vi "N-664 Test Panel.vi"() -> ()   [LabVIEW 2020]
uses:
  <vilib>/Instr/_visa.llb/VISA Configure Serial Port (Instr).vi
panel:
  out "Latest Error":errorcluster
  in  "COM Port":refnum<visa-resource-name>
  in  "Quit":bool
  out "Reply":string
  in  "Send Command":bool
  in  "Command":string
  # "*IDN? - Get device info"
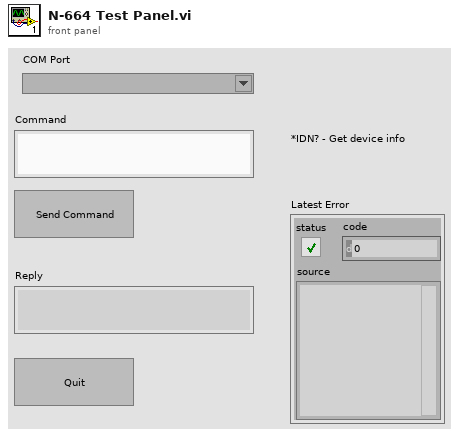
[diagram p1: front panel]
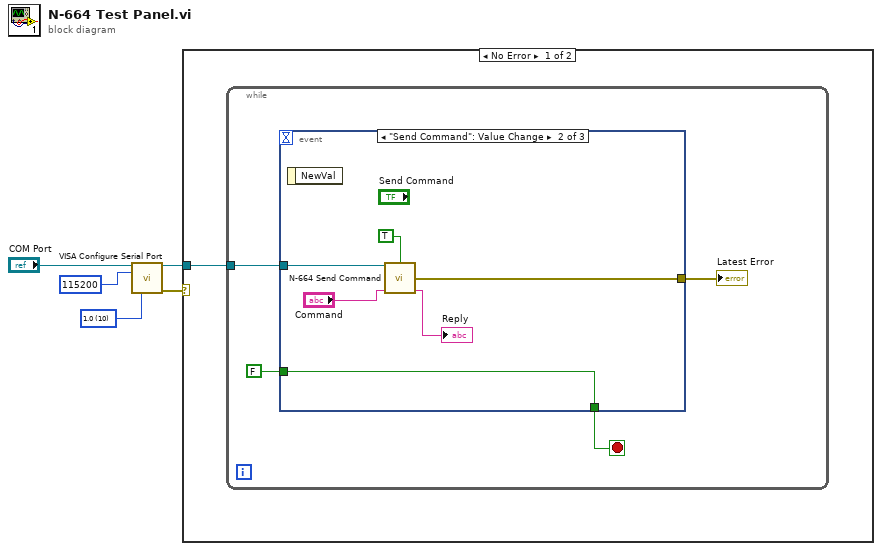
[diagram p0: block diagram]
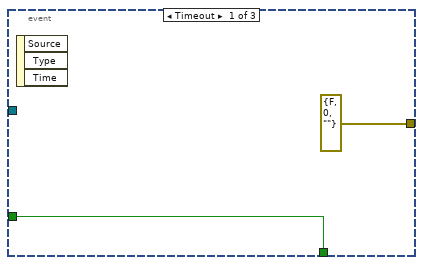
[diagram p2: hidden frame]
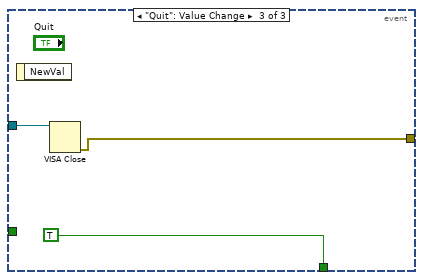
[diagram p3: hidden frame]
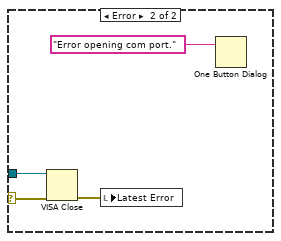
[diagram p4: hidden frame]
diagram:
  w5 = u16 10 items=["1.0"=10, "1.5"=15, "2.0"=20] ("stop bits (10: 1 bit)")
  n1 = call-poly "VISA Configure Serial Port"("VISA resource name"="COM Port", "baud rate (9600)"=u32 115200, "stop bits (10: 1 bit)"=w5) -> ("VISA resource name out"=w1:refnum<visa-resource-name>, "error out"=w2:errorcluster)  [unwired: 11 in]
  n2 = case shown="No Error" w2 {
    selector: w2 -> [_ w23]
    tunnel: w1 -> [w6 w24]
    frame No Error {
      n3 = while {
        tunnel: w6 -> [w8]
        stop <- w9 stop-if-true
        n4 = event shown="[1] \"Send Command\": Value Change" {
          selector: _ -> [_ _ _]
          dyn-events: _ -> [_ _ _]
          timeout: _ -> [_ _ _]
          tunnel: FALSE -> [w12 w18 _]
          tunnel: [w12 w18 TRUE] -> w9
          tunnel: w8 -> [_ w15 w20]
          tunnel: [errorcluster {"status"=FALSE, "code"=0, "source"=""} ("error out") w13 w19] -> w7
          event Timeout {
            n5 = event-data() -> ()  [unwired: 1 in, 3 out]
          }
          event "Send Command": Value Change {
            n6 = event-data() -> ()  [unwired: 1 in, 1 out]
            n7 = call "N-664 Send Command.vi"("VISA Ref"=w15, "Wait for Reply?"=TRUE, "Command"="Command") -> ("Error Out"=w13:errorcluster, "Response"=→"Reply":string)  [unwired: 10 in, 1 out]
          }
          event "Quit": Value Change {
            n8 = event-data() -> ()  [unwired: 1 in, 1 out]
            n9 = VISA Close(VISA resource name=w20) -> (error out=w19:errorcluster)  [unwired: 1 in]
          }
        }
        "Latest Error" <- w7
      }
    }
    frame Error {
      n10 = VISA Close(VISA resource name=w24, error in (no error)=w23) -> (error out=w22:errorcluster)
      n11 = local write "Latest Error"(w22) -> ()
      n12 = One Button Dialog(message="Error opening com port.") -> ()  [unwired: 1 in, 1 out]
    }
  }
